vi "read.vi"(8 "error in (no error)":errorcluster, 9 "Timeout":i32=25000, 10 "NumberOfBytes":i32, 11 "M1M3SAL in":refnum<class "M1M3SAL.lvclass">) -> (0 "error out":errorcluster, 1 "Timeout":bool, 2 "Data":u8[](array[numeric]), 3 "M1M3SAL out":refnum<class "M1M3SAL.lvclass">)   [LabVIEW 2016, in "M1M3Communicator.lvlib" / "M1M3SAL.lvclass"]
uses:
  M1M3SAL.lvclass
  M1M3SAL.lvclass/M1M3SAL.ctl
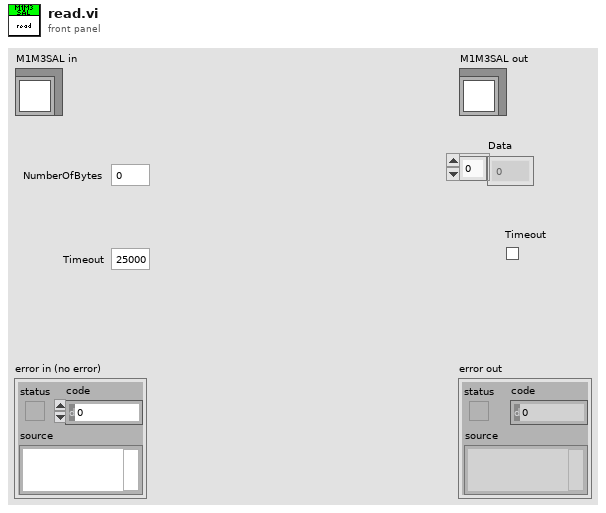
[diagram p1: front panel]
types:
  T1 = enum16{"Standard", "Buffered", "CRLF", "Immediate"}
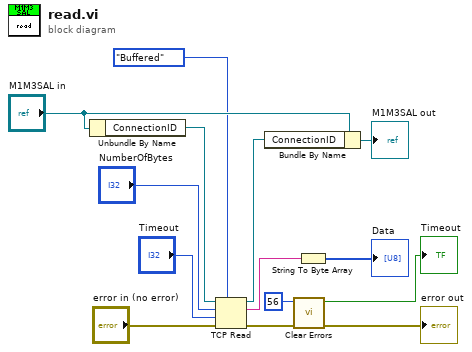
[diagram p0: block diagram]
diagram:
  n1 = Unbundle By Name("M1M3SAL in") -> ("ConnectionID"=w12:refnum<k5>)
  n2 = TCP Read(connection ID=w12, bytes to read="NumberOfBytes", error in (no error)="error in (no error)", 7:T1."Buffered" ("mode (standard)"), 9:"Timeout") -> (connection ID out=w11:refnum<k5>, data out=w9:string, error out=w2:errorcluster)
  n3 = Bundle By Name(cluster="M1M3SAL in", "ConnectionID"=w11) -> (→"M1M3SAL out":refnum<class "M1M3SAL.lvclass">)
  n4 = call <vilib>:"Clear Errors.vi"("error in (no error)"=w2, "specific error code to clear (0: all)"=56) -> ("error out"=→"error out":errorcluster, "specific error cleared?"=→"Timeout":bool)  [unwired: 4 in]
  n5 = String To Byte Array(string=w9) -> (unsigned byte array=→"Data":u8[])
